vi "EfieldOutStr.vi"(0 "noise?":bool, 2 "+ or -":bool=TRUE, 3 "badFormat?":bool, 4 "inputs_constant?":bool, 5 "Kv/m Amplitude":dbl format="%.2f", 6 "constant":dbl, 7 "seconds since 1Jan1904":dbl format="%.2f") -> (1 "data string":string)   [LabVIEW 2010]
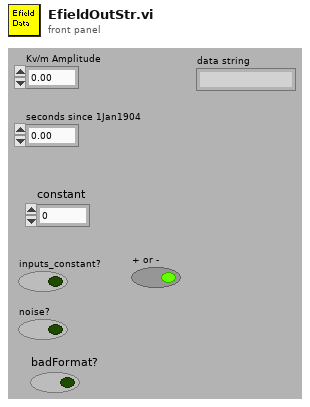
[diagram p1: front panel]
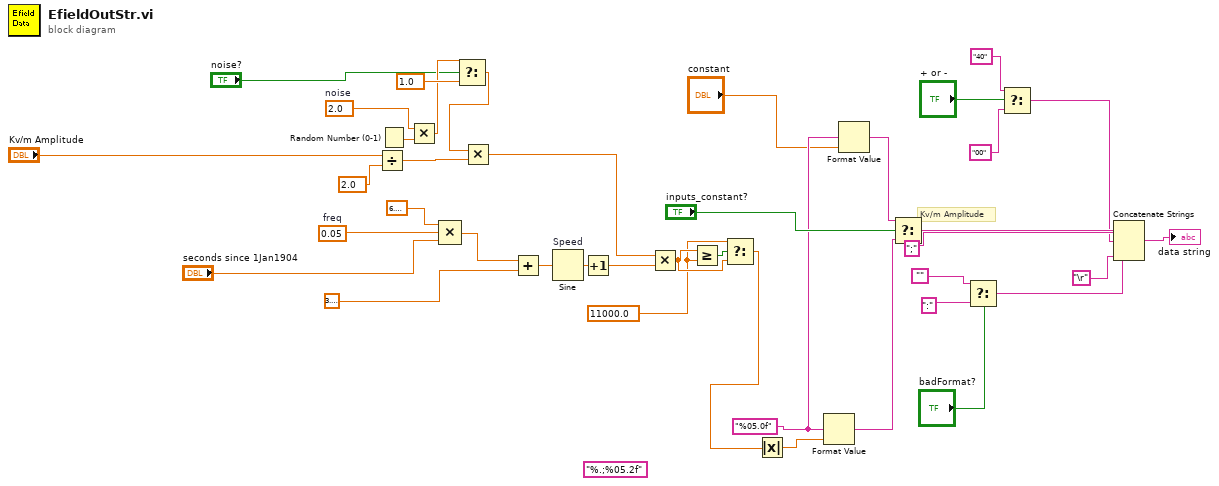
[diagram p0: block diagram]
diagram:
  (unwired) "%.;%05.2f" ("format string")
  w12 = "%05.0f" ("format string")
  w29 = 2.0  # noise
  w30 = 0.05  # freq
  w39 = 11000.0 ("y")
  # "Kv/m Amplitude"
  n1 = Divide(x="Kv/m Amplitude", y=2.0) -> (x/y=w35:dbl)
  n2 = Random Number (0-1)() -> (number: 0 to 1=w28:dbl)
  n3 = Multiply(x=w29, y=w28) -> (x*y=w19:dbl)
  n4 = Compound Arithmetic op=MULTIPLY(6.283185307179586, w30, "seconds since 1Jan1904") -> (w26:dbl)
  n5 = Select(t=w19, s="noise?", f=1.0) -> (s? t:f=w20:dbl)
  n6 = Multiply(x=w20, y=w35) -> (x*y=w37:dbl)
  n7 = Add(x=w26, y=3.141592653589793) -> (x+y=w25:dbl)
  n8 = Sine "Speed"(x=w25) -> (sin(x)=w24:dbl)
  n9 = Increment(x=w24) -> (x+1=w34:dbl)
  n10 = Multiply(x=w37, y=w34) -> (x*y=w40:dbl)
  n11 = Greater Or Equal?(x=w40, y=w39) -> (x >= y?=w38:bool)
  n12 = Select(t=w39, s=w38, f=w40) -> (s? t:f=w15:dbl)
  n13 = Absolute Value(x=w15) -> (abs(x)=w14:dbl)
  n14 = Format Value(format string=w12, value (0)=w14) -> (output string=w16:string)  [unwired: 1 in]
  n15 = Format Value(format string=w12, value (0)="constant") -> (output string=w10:string)  [unwired: 1 in]
  n16 = Select(t=w10, s="inputs_constant?", f=w16) -> (s? t:f=w17:string)
  n17 = Select(t="", s="badFormat?", f=":" ("string")) -> (s? t:f=w6:string)
  n18 = Select(t="40" ("string"), s="+ or -", f="00" ("string")) -> (s? t:f=w1:string)
  n19 = Concatenate Strings(w17, ";" ("string"), w1, w6, "\r") -> (→"data string":string)
